vi "AndorConvertErrCodeToMessage.vi"(8 "function return":u32) -> (0 "Element Return":cluster{i32, string})   [LabVIEW 2018, in "AndorOWN.lvlib"]
uses:
  AndorOWN.lvlib
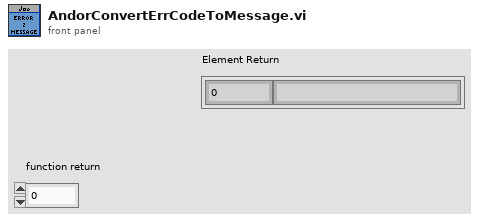
[diagram p1: front panel]
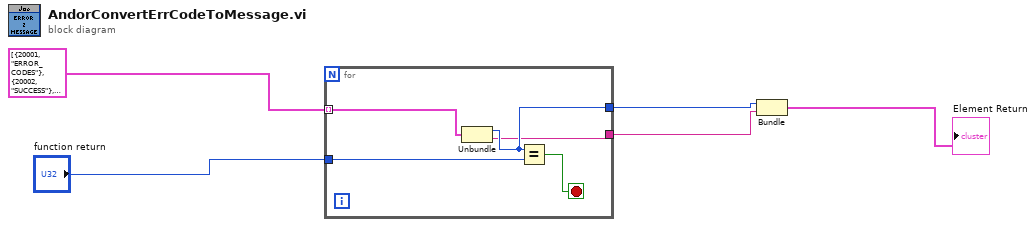
[diagram p0: block diagram]
diagram:
  n1 = for {
    tunnel: cluster{i32, string}[] [{20001, "ERROR_CODES"}, {20002, "SUCCESS"}, {20003, "VXDNOTINSTALLED"}, {20004, "ERROR_SCAN"}, {20005, "ERROR_CHECK_SUM"}, {20006, "ERROR_FILELOAD"}, {20007, "UNKNOWN_FUNCTION"}, {20008, "ERROR_VXD_INIT"}, {20009, "ERROR_ADDRESS"}, {20010, "ERROR_PAGELOCK"}, {20011, "ERROR_PAGE_UNLOCK"}, {20012, "ERROR_BOARDTEST"}, {20013, "ERROR_ACK"}, {20014, "ERROR_UP_FIFO"}, {20015, "ERROR_PATTERN"}, {20017, "ACQUISITION_ERRORS"}, {20018, "ACQ_BUFFER"}, {20019, "ACQ_DOWNFIFO_FULL"}, {20020, "PROC_UNKNOWN_INSTRUCTION"}, {20021, "ILLEGAL_OP_CODE"}, {20022, "KINETIC_TIME_NOT_MET"}, {20022, "KINETIC_TIME_NOT_MET"}, {20023, "ACCUM_TIME_NOT_MET"}, {20024, "NO_NEW_DATA"}, {20026, "SPOOLERROR"}, {20033, "TEMPERATURE_CODES"}, {20034, "TEMPERATURE_OFF"}, {20035, "TEMPERATURE_NOT_STABILIZED"}, {20036, "TEMPERATURE_STABILIZED"}, {20037, "TEMPERATURE_NOT_REACHED"}, {20038, "TEMPERATURE_OUT_RANGE"}, {20039, "TEMPERATURE_NOT_SUPPORTED"}, {20040, "TEMPERATURE_DRIFT"}, {20049, "GENERAL_ERRORS"}, {20050, "INVALID_AUX"}, {20051, "COF_NOTLOADED"}, {20052, "FPGAPROG"}, {20053, "FLEXERROR"}, {20054, "GPIBERROR"}, {20064, "DATATYPE"}, {20065, "DRIVER_ERRORS"}, {20066, "P1INVALID"}, {20067, "P2INVALID"}, {20068, "P3INVALID"}, {20069, "P4INVALID"}, {20070, "INIERROR"}, {20071, "COFERROR"}, {20072, "ACQUIRING"}, {20073, "IDLE"}, {20074, "TEMPCYCLE"}, {20075, "NOT_INITIALIZED"}, {20076, "P5INVALID"}, {20077, "P6INVALID"}, {20078, "INVALID_MODE"}, {20079, "INVALID_FILTER"}, {20080, "I2CERRORS"}, {20081, "DRV_I2CDEVNOTFOUND"}, {20082, "I2CTIMEOUT"}, {20083, "P7INVALID"}, {20089, "USBERROR"}, {20090, "IOCERROR"}, {20091, "NOT_SUPPORTED"}, {20093, "USB_INTERRUPT_ENDPOINT_ERROR"}, {20094, "RANDOM_TRACK_ERROR"}, {20095, "INVALID_TRIGGER_MODE"}, {20096, "LOAD_FIRMWARE_ERROR"}, {20097, "DIVIDE_BY_ZERO_ERROR"}, {20098, "INVALID_RINGEXPOSURES"}, {20099, "BINNING_ERROR"}, {20099, "BINNING_ERROR"}, {20100, "INVALID_AMPLIFIER"}, {20115, "ERROR_MAP"}, {20116, "ERROR_UNMAP"}, {20117, "ERROR_MDL"}, {20118, "ERROR_UNMDL"}, {20119, "ERROR_BUFFSIZE"}, {20121, "ERROR_NOHANDLE"}, {20130, "GATING_NOT_AVAILABLE"}, {20131, "FPGA_VOLTAGE_ERROR"}, {20990, "ERROR_NOCAMERA"}, {20991, "NOT_SUPPORTED"}, {20992, "NOT_AVAILABLE"}] ("Error Code Array") -> [w10] mode=indexing
    tunnel: "function return" -> [w9]
    tunnel: [w7] -> w4
    tunnel: [w6] -> w3
    stop <- w8 stop-if-true
    n2 = Unbundle(w10) -> (w7:i32, w6:string)
    n3 = Equal?(x=w7, y=w9) -> (x = y?=w8:bool)
  }
  n4 = Bundle(w4, w3) -> (→"Element Return":cluster{i32, string})  [unwired: 1 in]
